vi "SplashScreen.vi"(8 "error in (no error)":errorcluster) -> (0 "error out":errorcluster)   [LabVIEW 2013, in "main.lvlib"]
uses:
  main.lvlib
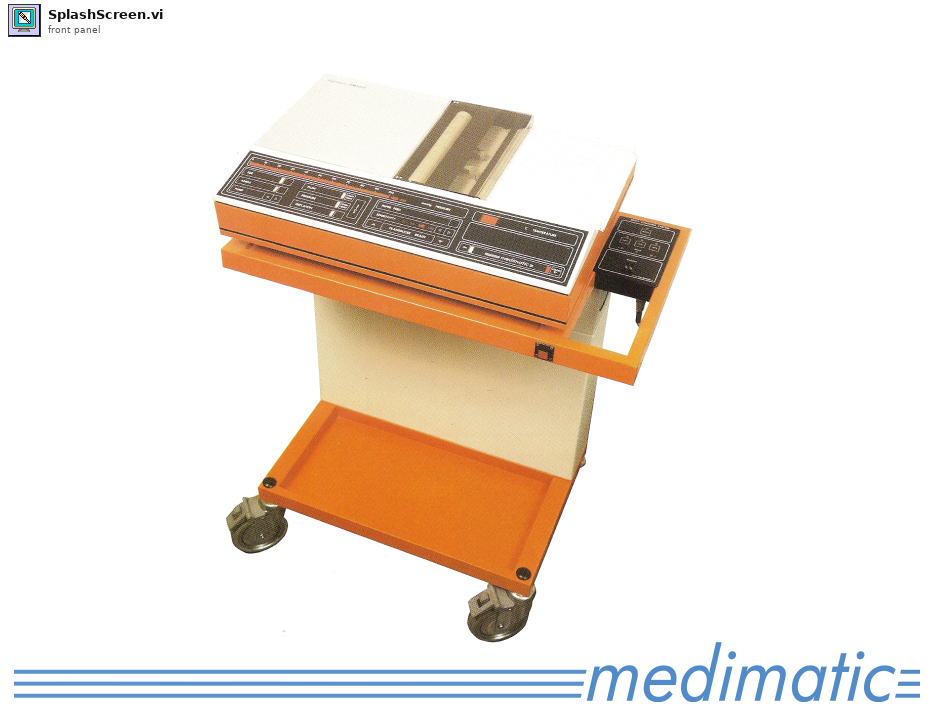
[diagram p1: front panel]
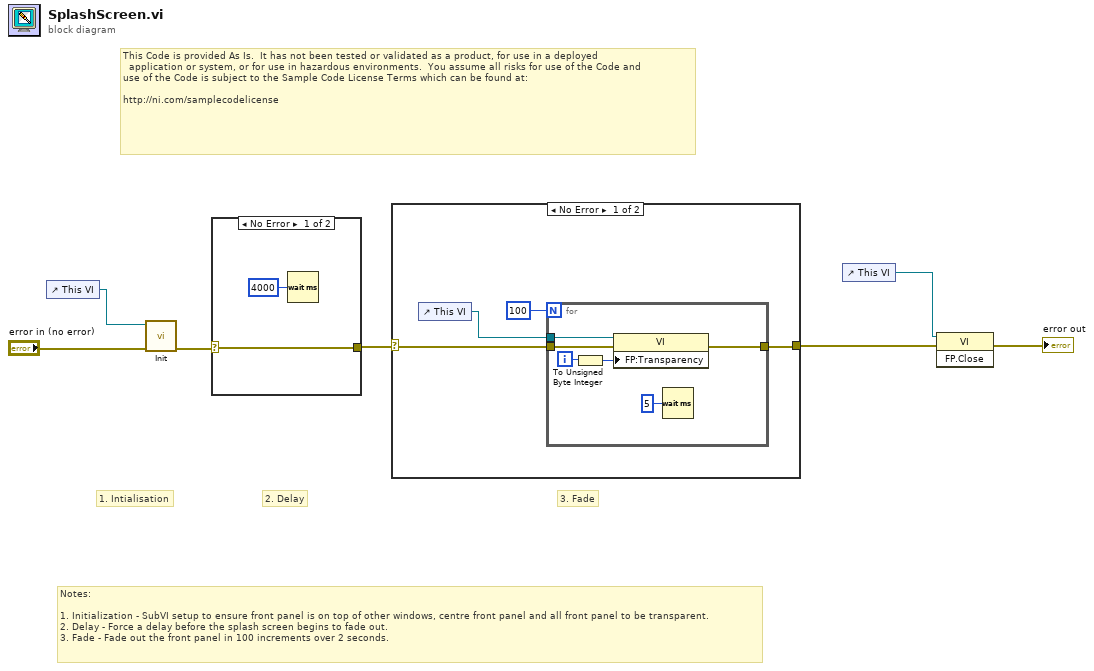
[diagram p0: block diagram]
diagram:
  # "This Code is provided As Is.  It has not been tested or validated as a product, for use in a deployed\n  application or system, or for use in hazardous environments.  You assume all risks for use of the Code and   \nuse of the Code is subject to the Sample Code License Terms which can be found at: \n\nhttp://ni.com/samplecodelicense"
  # "Notes:\n\n1. Initialization - SubVI setup to ensure front panel is on top of other windows, centre front panel and all front panel to be transparent.\n2. Delay - Force a delay before the splash screen begins to fade out.\n3. Fade - Fade out the front panel in 100 increments over 2 seconds."
  # "3. Fade"
  # "2. Delay"
  # "1. Intialisation"
  n1 = control-ref of="This VI"() -> (w5:refnum<vi>)
  n2 = call "Init.vi"("error in (no error)"="error in (no error)", "VI Refnum"=w5) -> ("error out"=w6:errorcluster)  [unwired: 9 in]
  n3 = case shown="No Error" w6 {
    selector: w6 -> [w9 w10]
    tunnel: [w9 w10] -> w7
    frame No Error {
      n4 = Wait (ms)(milliseconds to wait=u32 4000) -> ()  [unwired: 1 out]
    }
    frame Error {
    }
  }
  n5 = case shown="No Error" w7 {
    selector: w7 -> [w11 w21]
    tunnel: [w13 w21] -> w1
    frame No Error {
      n6 = control-ref of="This VI"() -> (w12:refnum<vi>)
      n7 = for {
        N: 100 -> [_]
        tunnel: [w18] -> w13
        tunnel: w12 -> [w16]
        tunnel: w11 -> [w15]
        i -> [w20]
        n8 = To Unsigned Byte Integer(number=w20) -> (unsigned 8bit integer=w19:u8)
        n9 = property class="VI"(reference=w16, error in=w15, "FP:Transparency"=w19) -> (error out=w18:errorcluster)  [unwired: 1 out]
        n10 = Wait (ms)(milliseconds to wait=u32 5) -> ()  [unwired: 1 out]
      }
    }
    frame Error {
    }
  }
  n11 = control-ref of="This VI"() -> (w3:refnum<vi>)
  n12 = invoke class="VI" method="FP.Close"(reference=w3, error in=w1) -> (error out=→"error out":errorcluster)  [unwired: 1 in, 2 out]
